vi "Keithley24xx_qMeash_FE.vi"(0 "c_VISA In":refnum<visa-resource-name>, 1 "MeasF In":string, 2 "b_VISA In":refnum<visa-resource-name>, 5 "max Level Ibase, A":dbl, 7 "b_Err In":errorcluster, 9 "min Level Ibase, A":dbl, 11 "c_Err In":errorcluster, 12 "Ic,A":dbl) -> (4 "b_VISA Out":refnum<visa-resource-name>, 6 "c_VISA Out":refnum<visa-resource-name>, 8 "hFE":dbl format="%#.3g", 10 "b_Err Out":errorcluster, 15 "c_VISA Out":errorcluster)   [LabVIEW 2014]
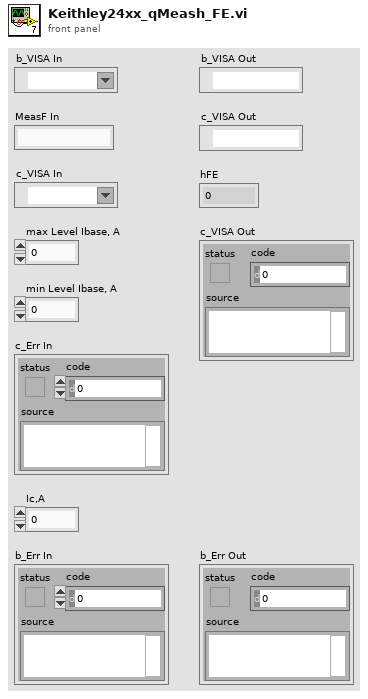
[diagram p1: front panel]
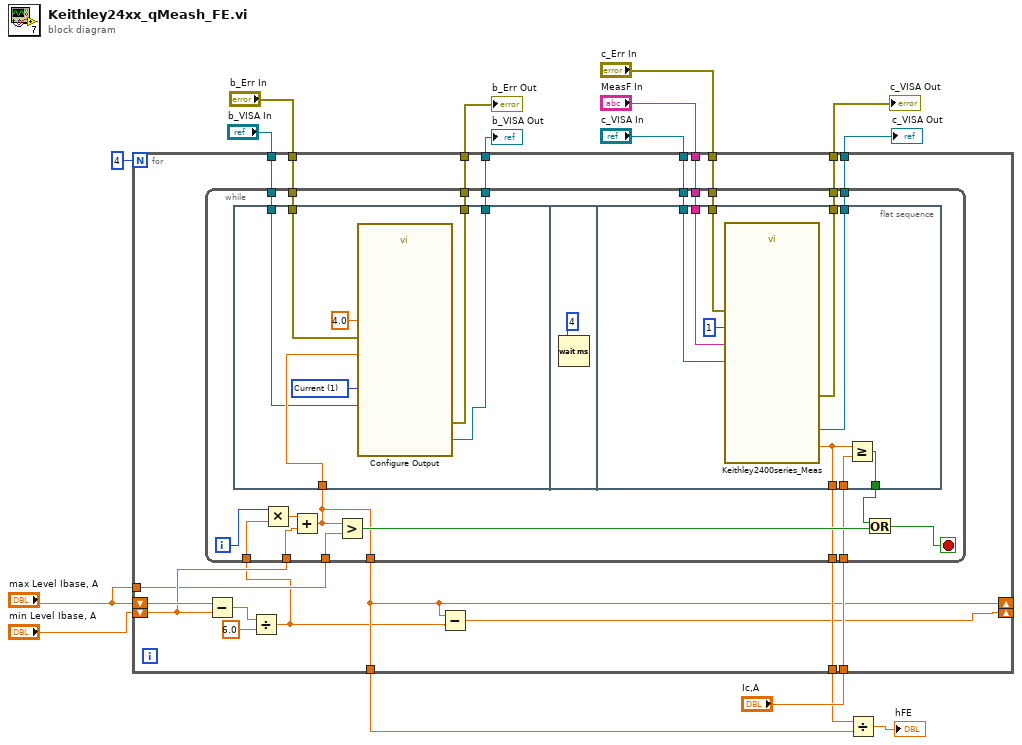
[diagram p0: block diagram]
diagram:
  n1 = for {
    N: 4 -> [_]
    tunnel: [w35] -> w1
    tunnel: "Ic,A" -> [w34]
    shift-right: [w28] -> _
    shift-left: "min Level Ibase, A" -> [w30]
    shift-right: [w27] -> _
    shift-left: "max Level Ibase, A" -> [w31]
    tunnel: [w27] -> w5
    tunnel: "max Level Ibase, A" -> [w29]
    tunnel: "c_Err In" -> [w25]
    tunnel: "MeasF In" -> [w24]
    tunnel: "c_VISA In" -> [w23]
    tunnel: [w22] -> w11
    tunnel: [w21] -> w12
    tunnel: "b_VISA In" -> [w20]
    tunnel: "b_Err In" -> [w19]
    tunnel: [w18] -> w15
    tunnel: [w17] -> w16
    n2 = Subtract(x=w31, y=w30) -> (x-y=w32:dbl)
    n3 = Divide(x=w32, y=6.0) -> (x/y=w26:dbl)
    n4 = while {
      tunnel: w26 -> [w51]
      tunnel: w30 -> [w50]
      tunnel: w29 -> [w49]
      tunnel: [w48] -> w35
      tunnel: [w47] -> w27
      tunnel: w34 -> [w46]
      tunnel: w25 -> [w44]
      tunnel: w24 -> [w43]
      tunnel: w23 -> [w42]
      tunnel: [w41] -> w22
      tunnel: [w40] -> w21
      tunnel: w20 -> [w39]
      tunnel: w19 -> [w38]
      tunnel: [w37] -> w18
      tunnel: [w36] -> w17
      i -> [w45]
      stop <- w52 stop-if-true
      n5 = flat-sequence {
        tunnel: w47 -> [w60]
        tunnel: w39 -> [w59]
        tunnel: w38 -> [w58]
        tunnel: [w57] -> w37
        tunnel: [w56] -> w36
        tunnel: [w71] -> w53
        tunnel: [w70] -> w48
        tunnel: w46 -> [w69]
        tunnel: w44 -> [w68]
        tunnel: w43 -> [w67]
        tunnel: w42 -> [w66]
        tunnel: [w65] -> w41
        tunnel: [w64] -> w40
        frame #0 {
          w62 = u16 1 items=["Voltage", "Current"] ("Source Mode  (0: Voltage)")
          n6 = call "Configure Output.vi"("Source Mode  (0: Voltage)"=w62, "error in (no error)"=w58, "Compliance  Level (0.1)"=4.0, "Output Level (0)"=w60, "VISA resource name"=w59) -> ("error out"=w57:errorcluster, "VISA resource name out"=w56:refnum<visa-resource-name>)  [unwired: 5 in]
        }
        frame #1 {
          n7 = Wait (ms)(milliseconds to wait=u32 4) -> ()  [unwired: 1 out]
        }
        frame #2 {
          n8 = call "Keithley2400series_Meas.vi"("MEAS:<f>"=w67, "error in (no error)"=w68, "MEAS mode, 0 Volt"=u16 1, "VISA resource name in"=w66) -> ("error out"=w65:errorcluster, "Замер"=w70:dbl, "VISA out"=w64:refnum<visa-resource-name>)  [unwired: 1 in, 1 out]
          n9 = Greater Or Equal?(x=w70, y=w69) -> (x >= y?=w71:bool)
        }
      }
      n10 = Multiply(x=w45, y=w51) -> (x*y=w55:dbl)
      n11 = Add(x=w55, y=w50) -> (x+y=w47:dbl)
      n12 = Greater?(x=w47, y=w49) -> (0:w54:bool)
      n13 = Or(x=w53, y=w54) -> (x .or. y?=w52:bool)
    }
    n14 = Subtract(x=w27, y=w26) -> (x-y=w28:dbl)
  }
  "c_VISA Out" <- w12
  "b_VISA Out" <- w16
  "b_Err Out" <- w15
  "c_VISA Out" <- w11
  n15 = Divide(x=w1, y=w5) -> (x/y=→"hFE":dbl)
